vi "Read Static Position.vi"(8 "error in (no error)":errorcluster, 11 "Static Overlay in":refnum<class "Static Overlay.lvclass">) -> (0 "error out":errorcluster, 2 "Static Position":T1, 3 "Static Overlay out":refnum<class "Static Overlay.lvclass">)   [LabVIEW 2014, in "Static Overlay.lvclass"]
uses:
  Static Overlay.lvclass
  Static Position.ctl
  Static Overlay.lvclass/Static Overlay.ctl
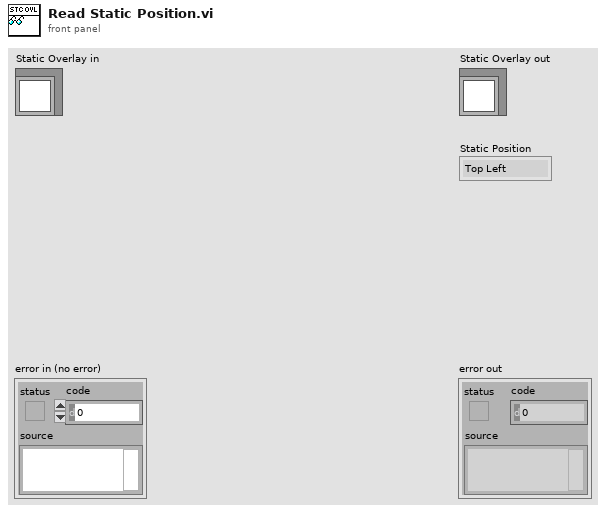
[diagram p1: front panel]
types:
  T1 = typedef "Static Overlay.lvclass/Static Position.ctl" = enum16{"Top Left", "Top Center", "Top Right", "Center", "Bottom Left", "Bottom Center", "Bottom Right"}
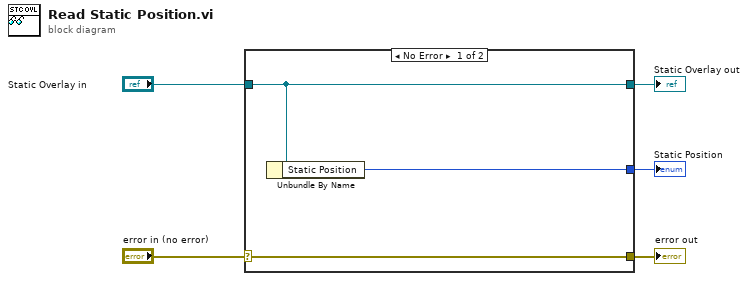
[diagram p0: block diagram]
diagram:
  n1 = case shown="No Error" "error in (no error)" {
    selector: "error in (no error)" -> [w8 w9]
    tunnel: [w8 w9] -> w4
    tunnel: [w7 w10] -> w2
    tunnel: "Static Overlay in" -> [w7 w10]
    tunnel: [w6 _] -> w1
    frame No Error {
      n2 = Unbundle By Name(w7) -> ("Static Position"=w6:T1)
    }
    frame Error {
    }
  }
  "error out" <- w4
  "Static Overlay out" <- w2
  "Static Position" <- w1
